vi "Create Route File.vi"() -> ()   [LabVIEW 2019]
uses:
  <vilib>/Utility/file.llb/Write Delimited Spreadsheet (string).vi
panel:
  out "File Path":path=path "C:/Users/bbrice_VM/Documents/LV Apps/LRMS/PPack_B Build/Config/File_Test.xls"
  in  "File Name (.csv)":string="File_Test"
  out "error out":errorcluster
  out "Route Specs":string[][](array[string])
  in  "Virtual Device Name":string="PPack_B_Test"
  in  "error in (no error)":errorcluster
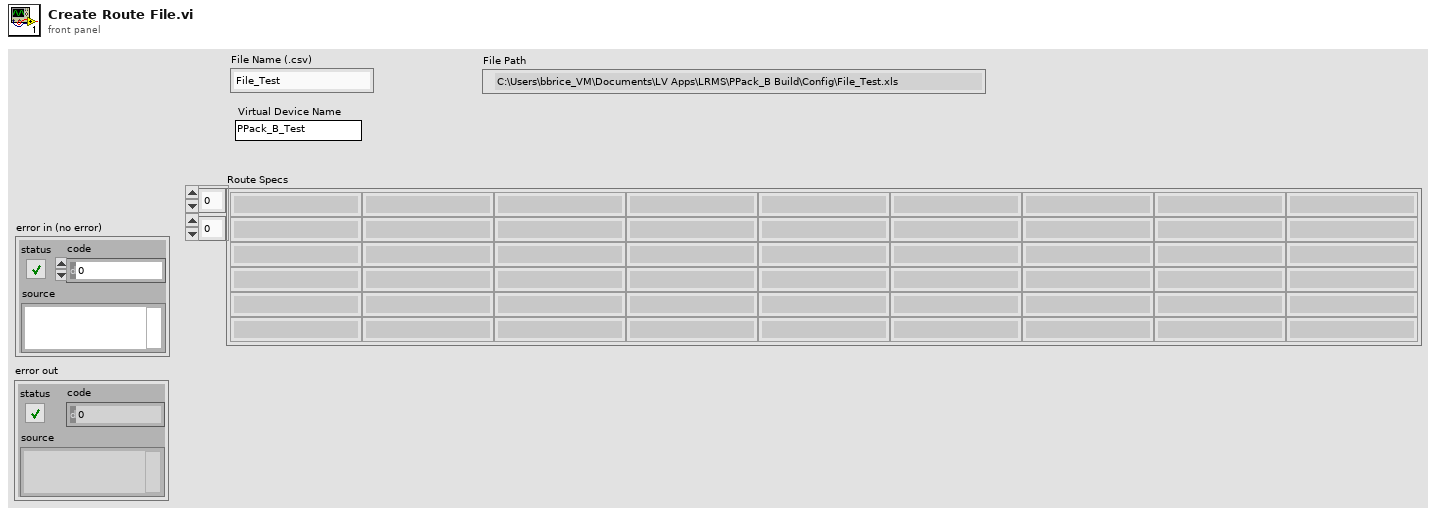
[diagram p1: front panel]
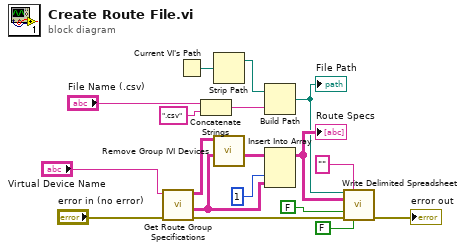
[diagram p0: block diagram]
diagram:
  n1 = call "Get Route Group Specifications.vi"("error in (no error)"="error in (no error)", "Virtual Device Name"="Virtual Device Name") -> ("error out"=w12:errorcluster, "IVI Names"=w13:string[][], "Specifications"=w16:string[][])  [unwired: 7 in]
  n2 = Current VI's Path() -> (path=w6:path)
  n3 = Concatenate Strings("File Name (.csv)", ".csv" ("string")) -> (w3:string)
  n4 = Strip Path(path=w6) -> (stripped path=w5:path)  [unwired: 1 out]
  n5 = call "Remove Group IVI Devices.vi"("IVI Names"=w13, "Specifications"=w16) -> ("Route Specs"=w15:string[][])  [unwired: 9 in]
  n6 = Build Path(base path=w5, name or relative path=w3) -> (appended path=w1:path)
  "File Path" <- w1
  n7 = Insert Into Array(array=w15, index (col)=1 ("disabled index (col)"), new element=w13) -> (w10:string[][])  [unwired: 1 in]
  "Route Specs" <- w10
  n8 = call-poly <vilib>:"Write Delimited Spreadsheet.vi"("file path (dialog if empty)"=w1, "format (%s)"="", "2D data"=w10, "append to file? (new file:F)"=FALSE, "error in (no error)"=w12, "transpose? (no:F)"=FALSE) -> ("error out"=→"error out":errorcluster)  [unwired: 8 in, 1 out]
